vi "lvversion keys.vi"() -> (3 "lv version keys":string[](array[string]))   [LabVIEW 2013]
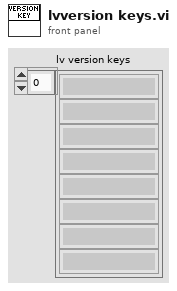
[diagram p1: front panel]
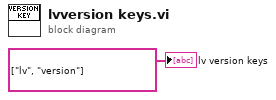
[diagram p0: block diagram]
diagram:
  "lv version keys" <- string[] ["lv", "version"] ("required keys")
